vi "문자열함수.vi"() -> ()   [LabVIEW 2014]
panel:
  out "이전 부분 문자열":string
  out "숫자":dbl
  out "부분 문자열":string
  out "길이":i32
  out "문자열 2":string
  in  "문자열":string
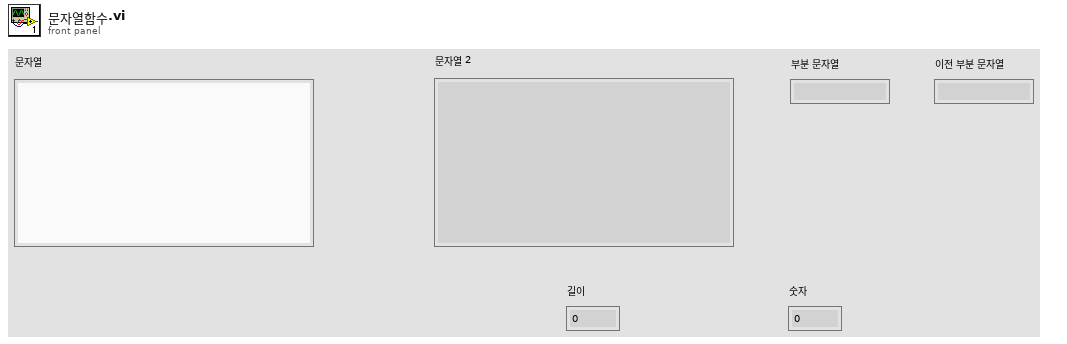
[diagram p1: front panel]
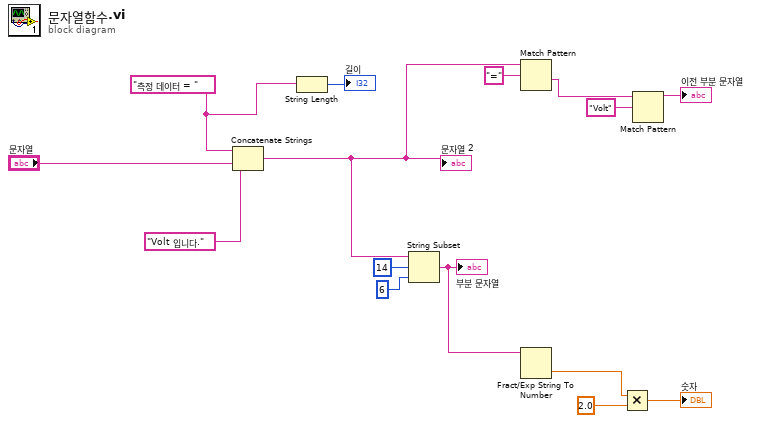
[diagram p0: block diagram]
diagram:
  w13 = "측정 데이터 = " ("문자열")
  n1 = Concatenate Strings(w13, "문자열", "Volt 입니다." ("문자열")) -> (w5:string)
  "문자열 2" <- w5
  n2 = String Length(string=w13) -> (length=→"길이":i32)
  n3 = String Subset(string=w5, offset (0)=14 ("오프셋(0)"), length (rest)=6 ("길이(나머지)")) -> (substring=w9:string)
  "부분 문자열" <- w9
  n4 = Match Pattern(string=w5, regular expression="=" ("정규식")) -> (after substring=w3:string)  [unwired: 1 in, 3 out]
  n5 = Fract/Exp String To Number(string=w9) -> (number=w8:dbl)  [unwired: 3 in, 1 out]
  n6 = Multiply(x=w8, y=2.0) -> (x*y=→"숫자":dbl)
  n7 = Match Pattern(string=w3, regular expression="Volt" ("정규식")) -> (before substring=→"이전 부분 문자열":string)  [unwired: 1 in, 3 out]
